vi "WriteDigitalLines.vi"(8 "error in (no error)":errorcluster, 10 "DigitalLines":tag[](array[tag]), 11 "NI Digital Output in":refnum<class "NI Digital Output.lvclass">) -> (0 "error out":errorcluster, 3 "NI Digital Output out":refnum<class "NI Digital Output.lvclass">)   [LabVIEW 2023, in "HardwareAbstractionLayer_LVOOP.lvlib" / "NI Digital Output.lvclass"]
doc: "This Passing Digital Lines"
uses:
  NI Digital Output.lvclass
  NI Digital Output.lvclass/NI Digital Output.ctl
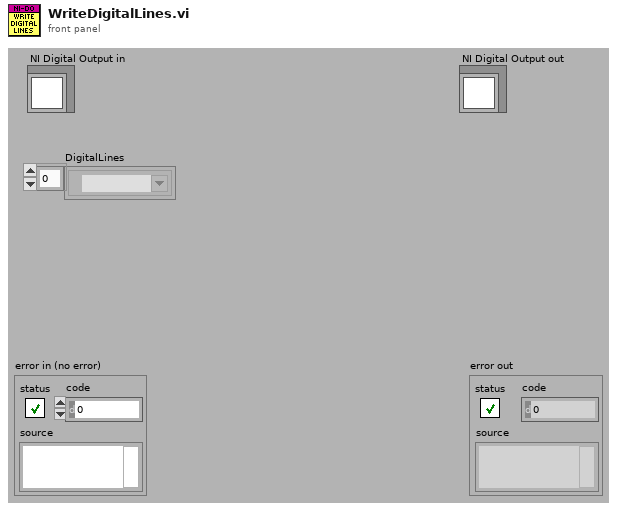
[diagram p1: front panel]
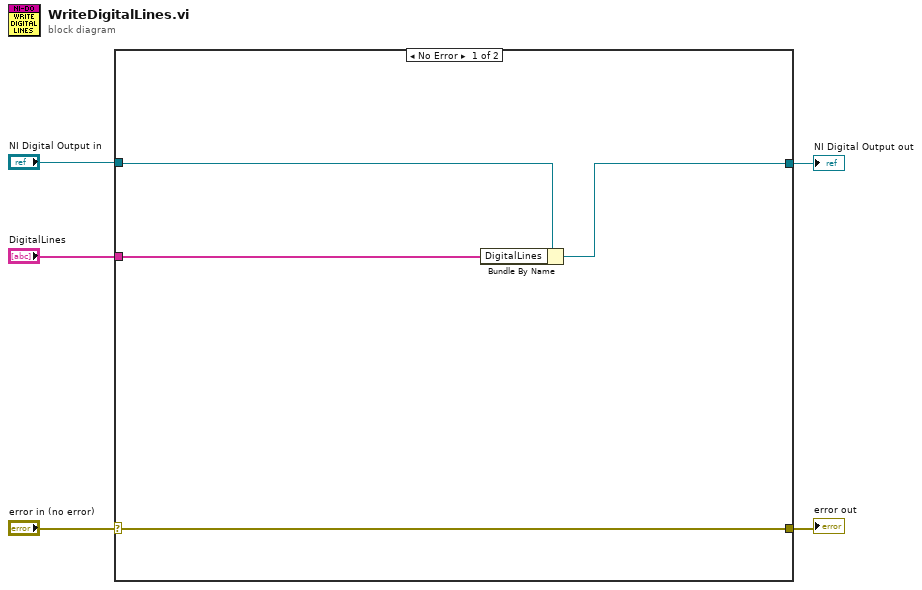
[diagram p0: block diagram]
diagram:
  n1 = case shown="No Error" "error in (no error)" {
    selector: "error in (no error)" -> [w8 w11]
    tunnel: [w8 w11] -> w4
    tunnel: [w6 w10] -> w2
    tunnel: "NI Digital Output in" -> [w7 w10]
    tunnel: "DigitalLines" -> [w9 _]
    frame No Error {
      n2 = Bundle By Name(cluster=w7, "DigitalLines"=w9) -> (w6:refnum<class "NI Digital Output.lvclass">)
    }
    frame Error {
    }
  }
  "error out" <- w4
  "NI Digital Output out" <- w2
